vi "Read Measurement Name.vi"(8 "error in":errorcluster, 11 "Input Channels in":refnum<class "Input Channels.lvclass">) -> (0 "error out":errorcluster, 2 "Measurement Name":string, 3 "Input Channels out":refnum<class "Input Channels.lvclass">)   [LabVIEW 2020, in "Plugin.lvlib" / "Input Channels.lvclass"]
doc: "Reads measurement name."
uses:
  Input Channels.lvclass
panel:
  out "length":i32
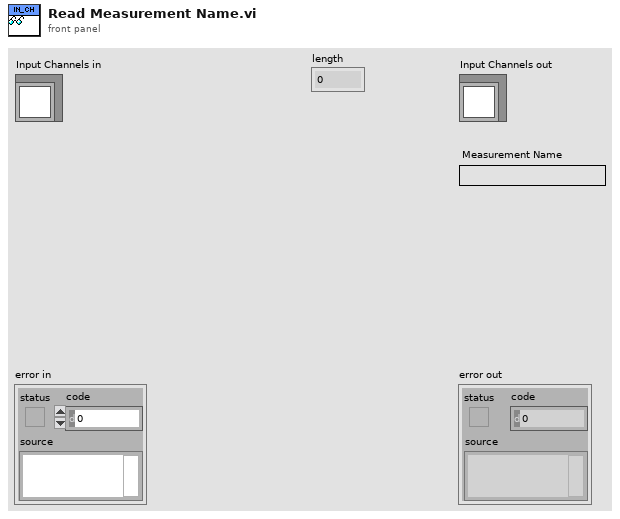
[diagram p1: front panel]
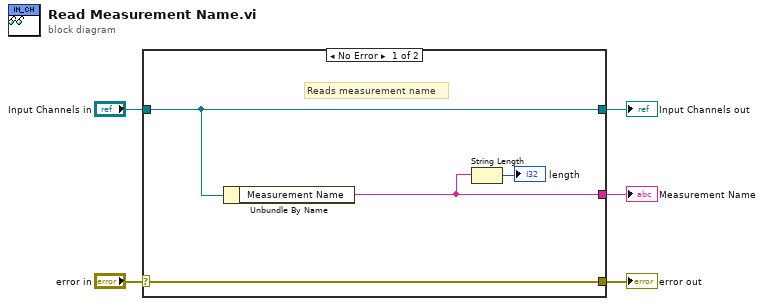
[diagram p0: block diagram]
diagram:
  n1 = case shown="No Error" "error in" {
    selector: "error in" -> [w9 w10]
    tunnel: [w9 w10] -> w4
    tunnel: [w8 w11] -> w2
    tunnel: "Input Channels in" -> [w8 w11]
    tunnel: [w7 _] -> w1
    frame No Error {
      # "Reads measurement name"
      n2 = Unbundle By Name(w8) -> ("Measurement Name"=w7:string)
      n3 = String Length(string=w7) -> (length=→"length":i32)
    }
    frame Error {
    }
  }
  "error out" <- w4
  "Input Channels out" <- w2
  "Measurement Name" <- w1
